vi "Proyecto Final_Topicos.vi"() -> ()   [LabVIEW 2020]
uses:
  <vilib>/Instr/_visa.llb/VISA Configure Serial Port (Instr).vi
  <vilib>/vision/NI_Vision_Development_Module.lvlib
panel:
  out "Buffer Completo":string
  out "Number of Particles":i32
  out "Particle Reports (Real-World)":T1(array[cluster]) {"Orientation" format="%.2f"; "Dimensions"."Height" format="%.2f"; "Dimensions"."Width" format="%.2f"; "Center of Mass"."Y" format="%.2f"; "Center of Mass"."X" format="%.2f"; "Bounding Rect"."Bottom" format="%.2f"; "Bounding Rect"."Right" format="%.2f"; "Bounding Rect"."Top" format="%.2f"; "Bounding Rect"."Left" format="%.2f"; "Number of Holes" format="%.2f"; "Area" format="%.2f"}
  in  "Tab Control":T2(tab)
  out "Original":T3(plugin-control) caption="Original Image"
  out "Threshold":T3(plugin-control) caption="Threshold Image"
  out "Fill Hole and Reject Border":T3(plugin-control) caption="Reject Border and Fill Holes"
  out "ROJO":bool
  out "VERDE":bool
  out "AMBAR":bool
  out "Área de particulas":T4(graph)
  out "Área de particualas total":dbl
  in  "name or relative path":path=path "C:/Users/axel2/Downloads/Proyecto Topicos/mexico_tmo_2013066_lrg.jpg"
  out "Valores House Keeping":T5
  out "Señales Analógicas":dynamicdata(graph)
  out "Señales Digitales":dynamicdata(graph)
  out "Buffer Filtrado":string
  out "error out":errorcluster
  in  "error in (no error)":errorcluster
  out "LISTO?":bool=TRUE
  in  "stop":bool
  in  "Comando":T6(ring)
  in  "Decisión":bool
  in  "VISA resource":refnum<visa-resource-name>="COM4"
  # "Variables del Satélite GXIBA"
  # "Comunicación con Satélite"
  # "Procesamiento de Riesgo Volcánico"
  # "SEMÁFORO VOLCÁNICO"
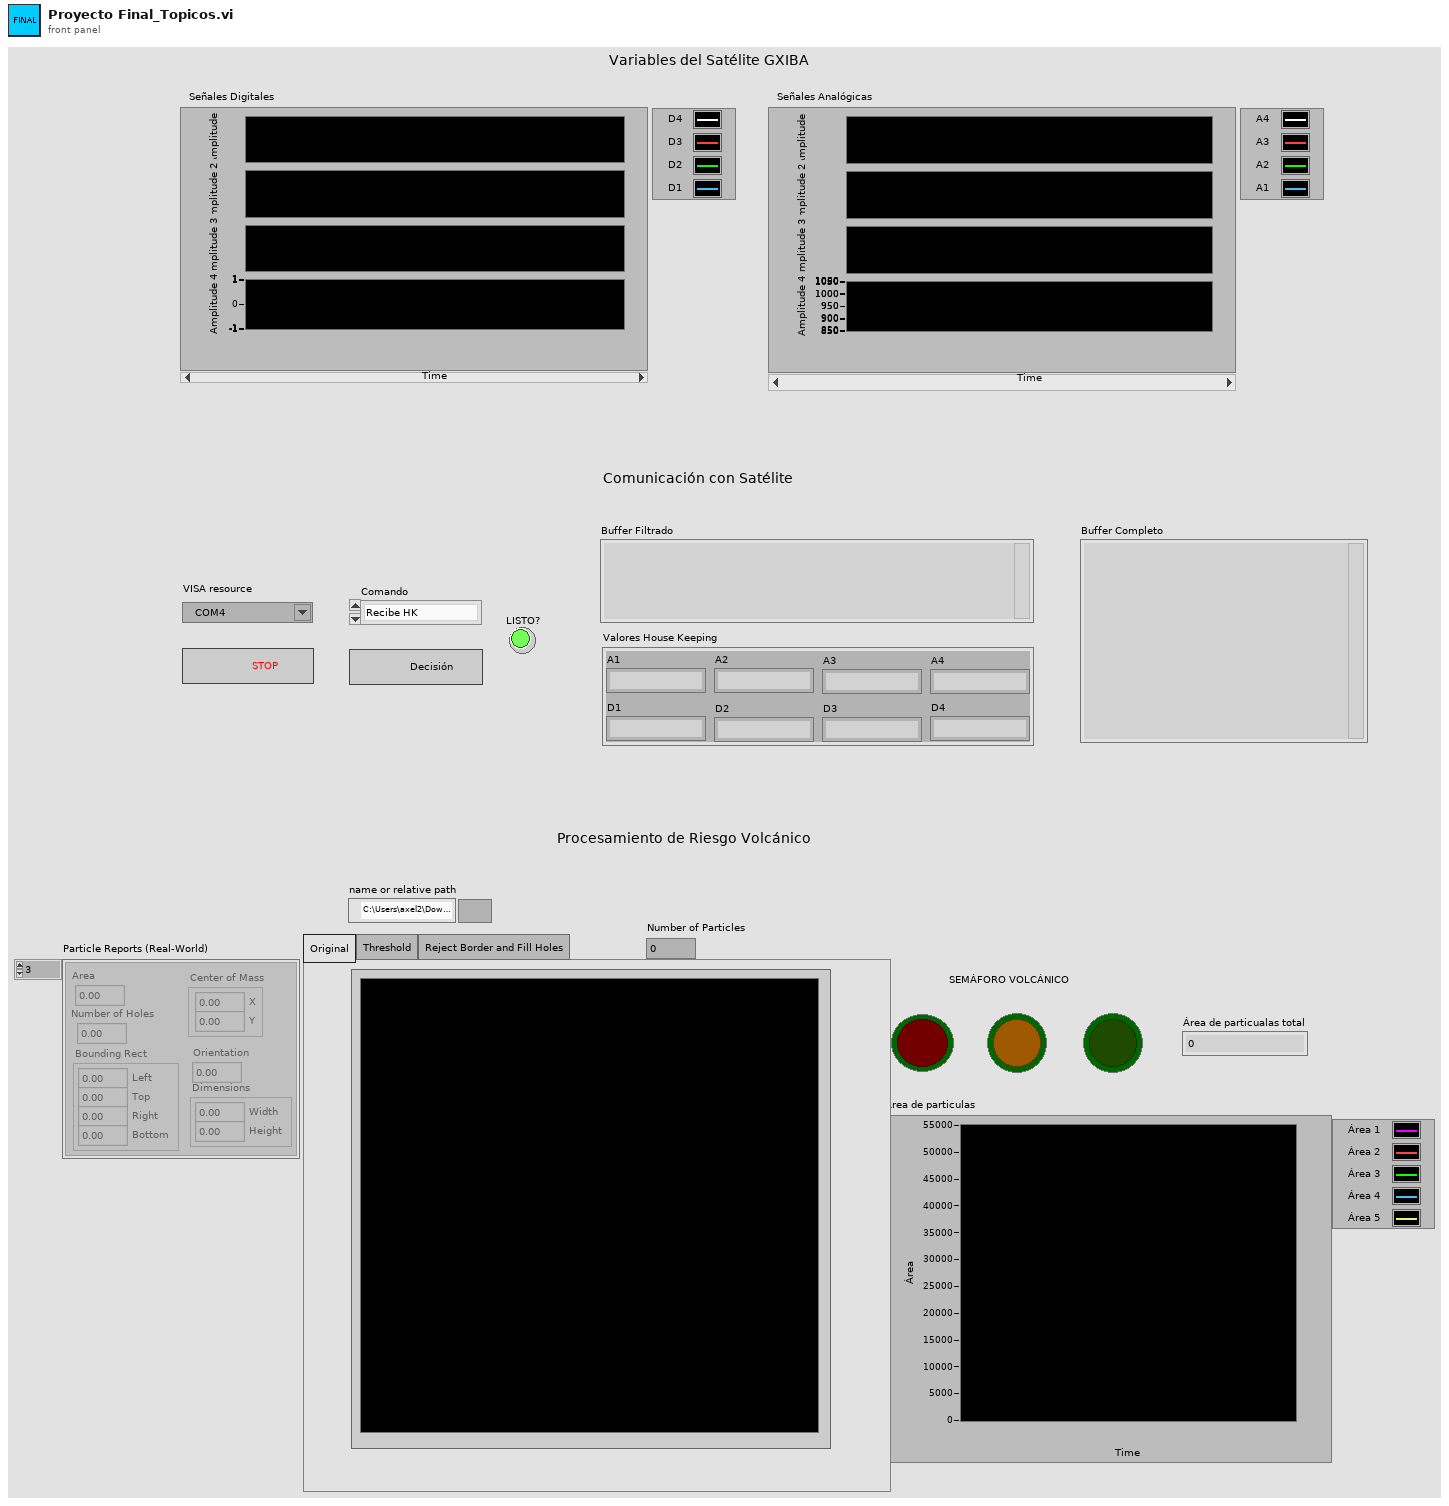
[diagram p1: front panel]
types:
  T1 = cluster{"Area":dbl, "Number of Holes":dbl, "Bounding Rect":cluster{"Left":dbl, "Top":dbl, "Right":dbl, "Bottom":dbl}, "Center of Mass":cluster{"X":dbl, "Y":dbl}, "Orientation":dbl, "Dimensions":cluster{"Width":dbl, "Height":dbl}}[]
  T2 = enum32{"Original", "Threshold", "Reject Border and Fill Holes"}
  T3 = typedef "IMAQ Image.ctl" = refnum<image>
  T4 = cluster{"Area":dbl, "Area":dbl, "Area":dbl, "Area":dbl, "Area":dbl}
  T5 = cluster{"A1":string, "A2":string, "A3":string, "A4":string, "D1":string, "D2":string, "D3":string, "D4":string}
  T6 = enum16{"Recibe HK", "Act Fecha", "Parametros", "Reset", "Stop"}
  T7 = typedef "Image Type" = u32
  T8 = cluster{"Particle Reports (Real-World)  [0]":cluster{"Area":dbl, "Number of Holes":dbl, "Bounding Rect":cluster{"Left":dbl, "Top":dbl, "Right":dbl, "Bottom":dbl}, "Center of Mass":cluster{"X":dbl, "Y":dbl}, "Orientation":dbl, "Dimensions":cluster{"Width":dbl, "Height":dbl}}, "Particle Reports (Real-World)  [1]":cluster{"Area":dbl, "Number of Holes":dbl, "Bounding Rect":cluster{"Left":dbl, "Top":dbl, "Right":dbl, "Bottom":dbl}, "Center of Mass":cluster{"X":dbl, "Y":dbl}, "Orientation":dbl, "Dimensions":cluster{"Width":dbl, "Height":dbl}}, "Particle Reports (Real-World)  [2]":cluster{"Area":dbl, "Number of Holes":dbl, "Bounding Rect":cluster{"Left":dbl, "Top":dbl, "Right":dbl, "Bottom":dbl}, "Center of Mass":cluster{"X":dbl, "Y":dbl}, "Orientation":dbl, "Dimensions":cluster{"Width":dbl, "Height":dbl}}, "Particle Reports (Real-World)  [3]":cluster{"Area":dbl, "Number of Holes":dbl, "Bounding Rect":cluster{"Left":dbl, "Top":dbl, "Right":dbl, "Bottom":dbl}, "Center of Mass":cluster{"X":dbl, "Y":dbl}, "Orientation":dbl, "Dimensions":cluster{"Width":dbl, "Height":dbl}}, "Particle Reports (Real-World)  [4]":cluster{"Area":dbl, "Number of Holes":dbl, "Bounding Rect":cluster{"Left":dbl, "Top":dbl, "Right":dbl, "Bottom":dbl}, "Center of Mass":cluster{"X":dbl, "Y":dbl}, "Orientation":dbl, "Dimensions":cluster{"Width":dbl, "Height":dbl}}, "Particle Reports (Real-World)  [5]":cluster{"Area":dbl, "Number of Holes":dbl, "Bounding Rect":cluster{"Left":dbl, "Top":dbl, "Right":dbl, "Bottom":dbl}, "Center of Mass":cluster{"X":dbl, "Y":dbl}, "Orientation":dbl, "Dimensions":cluster{"Width":dbl, "Height":dbl}}, "Particle Reports (Real-World)  [6]":cluster{"Area":dbl, "Number of Holes":dbl, "Bounding Rect":cluster{"Left":dbl, "Top":dbl, "Right":dbl, "Bottom":dbl}, "Center of Mass":cluster{"X":dbl, "Y":dbl}, "Orientation":dbl, "Dimensions":cluster{"Width":dbl, "Height":dbl}}, "Particle Reports (Real-World)  [7]":cluster{"Area":dbl, "Number of Holes":dbl, "Bounding Rect":cluster{"Left":dbl, "Top":dbl, "Right":dbl, "Bottom":dbl}, "Center of Mass":cluster{"X":dbl, "Y":dbl}, "Orientation":dbl, "Dimensions":cluster{"Width":dbl, "Height":dbl}}, "Particle Reports (Real-World)  [8]":cluster{"Area":dbl, "Number of Holes":dbl, "Bounding Rect":cluster{"Left":dbl, "Top":dbl, "Right":dbl, "Bottom":dbl}, "Center of Mass":cluster{"X":dbl, "Y":dbl}, "Orientation":dbl, "Dimensions":cluster{"Width":dbl, "Height":dbl}}}
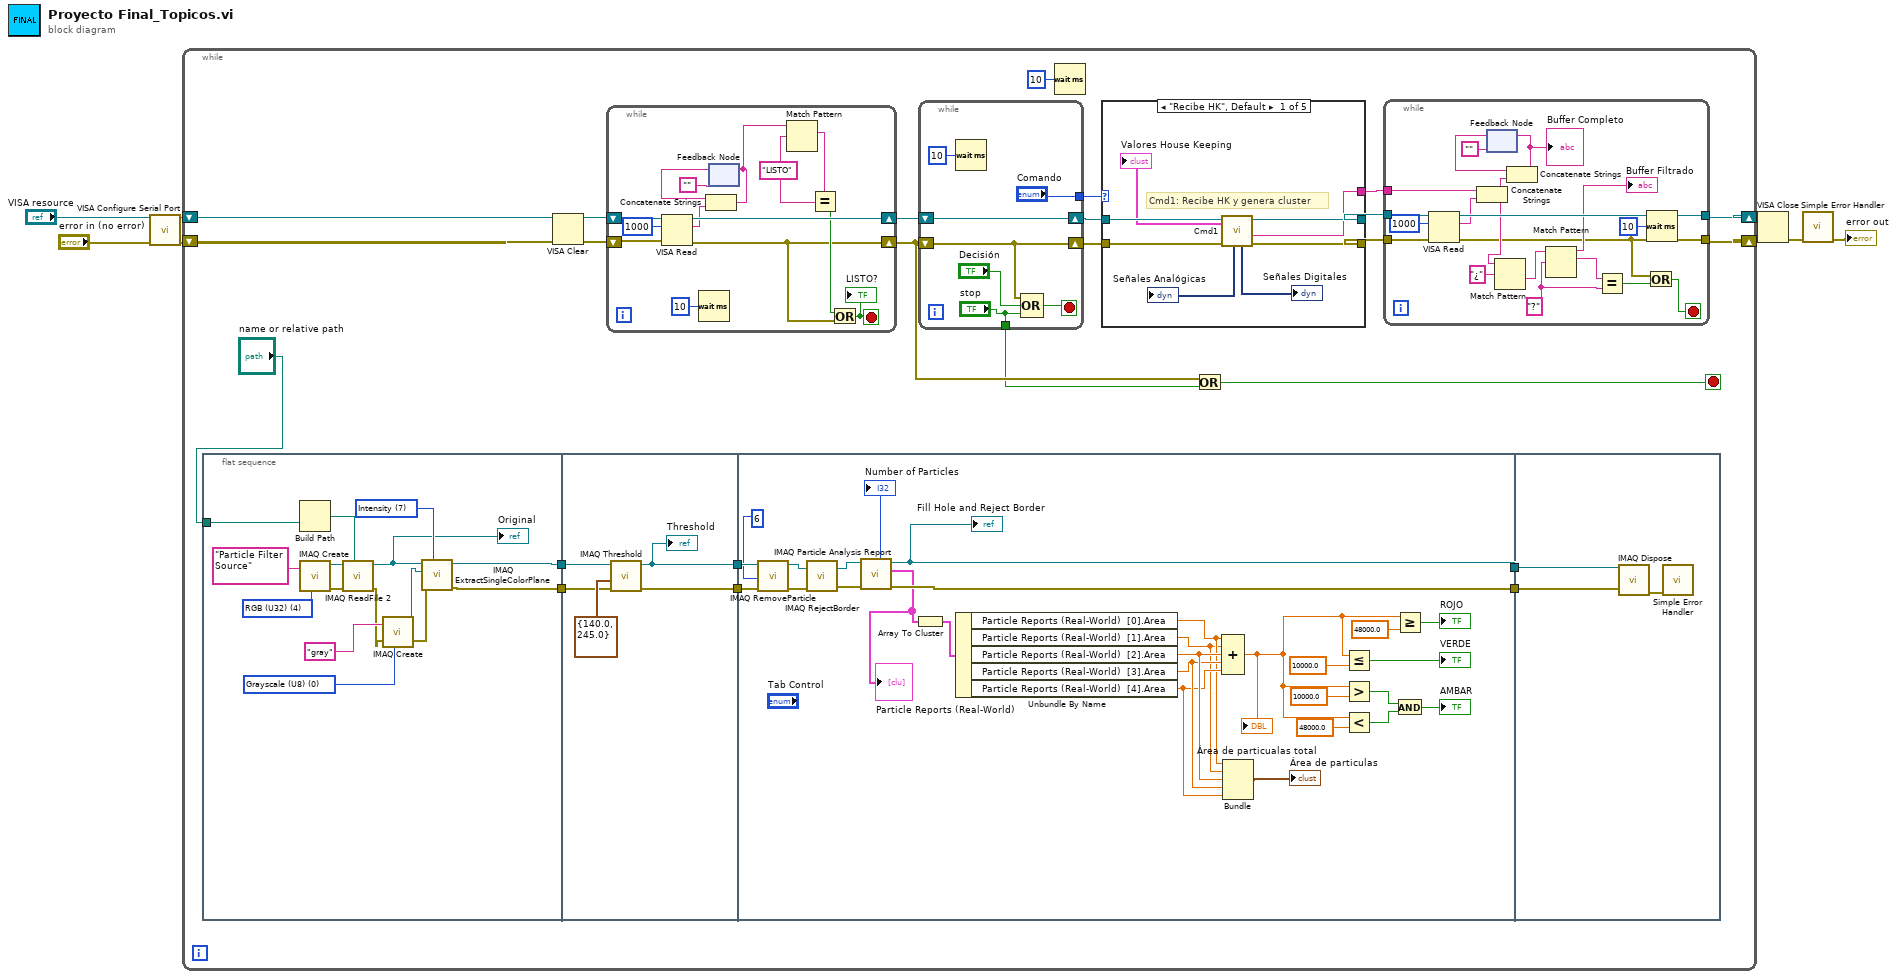
[diagram p0: block diagram]
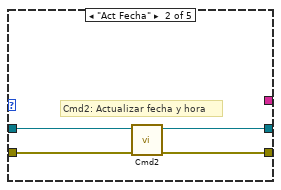
[diagram p2: hidden frame]
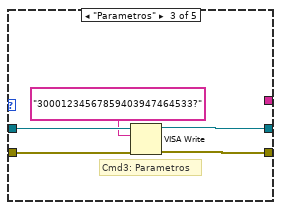
[diagram p3: hidden frame]
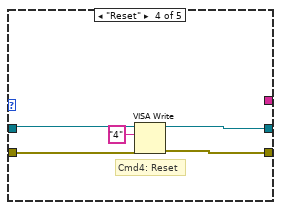
[diagram p4: hidden frame]
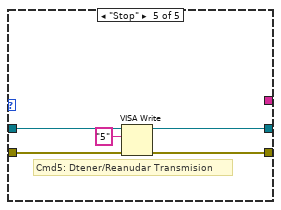
[diagram p5: hidden frame]
diagram:
  n1 = call-poly "VISA Configure Serial Port"("VISA resource name"="VISA resource", "error in (no error)"="error in (no error)") -> ("VISA resource name out"=w2:refnum<visa-resource-name>, "error out"=w1:errorcluster)  [unwired: 12 in]
  n2 = while {
    shift-right: [w19] -> w5
    shift-left: w1 -> [w25]
    shift-right: [w20] -> w6
    shift-left: w2 -> [w27]
    stop <- w28 stop-if-true
    n3 = flat-sequence {
      tunnel: [w35] -> w15
      tunnel: [w42] -> w14
      tunnel: "name or relative path" -> [w33]
      tunnel: [w50] -> w13
      tunnel: [w51] -> w12
      tunnel: w15 -> [w49]
      tunnel: w14 -> [w48]
      tunnel: w13 -> [w80]
      tunnel: w12 -> [w79]
      tunnel: [w54] -> w11
      tunnel: [w73] -> w10
      tunnel: w11 -> [w82]
      tunnel: w10 -> [w81]
      frame #0 {
        w39 = T7 0 items=["Grayscale (U8)", "Grayscale (I16)", "Grayscale (SGL)", "Complex (CSG)", "RGB (U32)", "HSL (U32)", "RGB (U64)", "Grayscale (U16)"] ("Image Type")
        w41 = 7 items=["Red", "Green", "Blue", "Hue", "Saturation", "Luminance", "Value", "Intensity"] ("Color Plane")
        w43 = T7 4 items=["Grayscale (U8)", "Grayscale (I16)", "Grayscale (SGL)", "Complex (CSG)", "RGB (U32)", "HSL (U32)", "RGB (U64)", "Grayscale (U16)"] ("Image Type")
        n4 = Build Path(name or relative path=w33) -> (appended path=w47:path)  [unwired: 1 in]
        n5 = call "IMAQ Create"("Image Name"="Particle Filter Source", "Image Type"=w43) -> ("New Image"=w45:T3, "error out"=w44:errorcluster)  [unwired: 3 in]
        n6 = call "IMAQ ReadFile 2"("File Path"=w47, "error in (no error)"=w44, "Image"=w45) -> ("error out"=w37:errorcluster, "Image Out"=w34:T3)  [unwired: 4 in, 3 out]
        "Original" <- w34
        n7 = call "IMAQ Create"("Image Name"="gray", "Image Type"=w39, "error in (no error)"=w37) -> ("New Image"=w40:T3, "error out"=w36:errorcluster)  [unwired: 2 in]
        n8 = call "IMAQ ExtractSingleColorPlane"("Color Plane"=w41, "error in (no error)"=w36, "Image Dst"=w40, "Image Src"=w34) -> ("error out"=w42:errorcluster, "Image Dst Out"=w35:T3)  [unwired: 6 in]
      }
      frame #1 {
        n9 = call "IMAQ Threshold"("error in (no error)"=w48, "Range"=cluster{"Lower value":sgl, "Upper value":sgl} {"Lower value"=140.0, "Upper value"=245.0}, "Image Src"=w49) -> ("error out"=w51:errorcluster, "Image Dst Out"=w50:T3)  [unwired: 7 in]
        "Threshold" <- w50
      }
      frame #2 {
        n10 = call "IMAQ RemoveParticle"("error in (no error)"=w79, "Number of Erosion"=6, "Image Src"=w80) -> ("error out"=w77:errorcluster, "Image Dst Out"=w78:T3)  [unwired: 7 in]
        n11 = call "IMAQ RejectBorder"("error in (no error)"=w77, "Image Src"=w78) -> ("error out"=w74:errorcluster, "Image Dst Out"=w75:T3)  [unwired: 4 in]
        n12 = call "IMAQ Particle Analysis Report"("error in (no error)"=w74, "Image"=w75) -> ("error out"=w73:errorcluster, "Particle Reports (Real-World)"=w53:T1, "Image Out (duplicate)"=w54:T3, "Number of Particles"=→"Number of Particles":i32)  [unwired: 6 out]
        "Fill Hole and Reject Border" <- w54
        "Particle Reports (Real-World)" <- w53
        n13 = Array To Cluster(array=w53) -> (cluster=w72:T8)
        n14 = Unbundle By Name(w72) -> ("Particle Reports (Real-World)  [0].Area"=w58:dbl, "Particle Reports (Real-World)  [1].Area"=w57:dbl, "Particle Reports (Real-World)  [2].Area"=w61:dbl, "Particle Reports (Real-World)  [3].Area"=w60:dbl, "Particle Reports (Real-World)  [4].Area"=w59:dbl)
        n15 = Compound Arithmetic op=ADD(w58, w57, w61, w60, w59) -> (w62:dbl)
        "Área de particualas total" <- w62
        n16 = Bundle("Area"=w58, "Area"=w57, "Area"=w61, "Area"=w60, "Area"=w59) -> (→"Área de particulas":T4)  [unwired: 1 in]
        n17 = Less Or Equal?(x=w62, y=10000.0) -> (x <= y?=→"VERDE":bool)
        n18 = Greater?(x=w62, y=10000.0) -> (0:w69:bool)
        n19 = Less?(x=w62, y=48000.0) -> (x < y?=w68:bool)
        n20 = Greater Or Equal?(x=w62, y=48000.0) -> (x >= y?=→"ROJO":bool)
        n21 = And(x=w69, y=w68) -> (x .and. y?=→"AMBAR":bool)
      }
      frame #3 {
        n22 = call "IMAQ Dispose"("Image"=w82, "error in (no error)"=w81) -> ("error out"=w83:errorcluster)  [unwired: 4 in]
        n23 = call <vilib>:"Simple Error Handler.vi"("error in (no error)"=w83) -> ()  [unwired: 4 in, 5 out]
      }
    }
    n24 = VISA Clear(VISA resource name=w27, error in (no error)=w25) -> (VISA resource name out=w26:refnum<visa-resource-name>, error out=w24:errorcluster)
    n25 = while {
      shift-right: [w138] -> w18
      shift-left: w24 -> [w149]
      shift-right: [w147] -> w30
      shift-left: w26 -> [w150]
      stop <- w137 stop-if-true
      w140 = "LISTO" ("regular expression")
      n26 = VISA Read(VISA resource name=w150, byte count=u32 1000, error in (no error)=w149) -> (VISA resource name out=w147:refnum<visa-resource-name>, read buffer=w146:string, error out=w138:errorcluster)  [unwired: 1 out]
      n27 = Wait (ms)(milliseconds to wait=u32 10) -> ()  [unwired: 1 out]
      n28 = feedback #1("") -> (w145:string)
      n29 = Concatenate Strings(w145, w146) -> (w142:string)
      n30 = feedback-in #1(w142) -> ()
      n31 = Match Pattern(string=w142, regular expression=w140) -> (match substring=w141:string)  [unwired: 1 in, 3 out]
      n32 = Equal?(x=w141, y=w140) -> (x = y?=w139:bool)
      n33 = Or(x=w139, y=w138) -> (x .or. y?=w137:bool)
      "LISTO?" <- w137
    }
    n34 = while {
      tunnel: ["Comando"] -> w32
      shift-right: [w108] -> w31
      shift-left: w30 -> [w108]
      shift-right: [w105] -> w29
      shift-left: w18 -> [w105]
      tunnel: ["stop"] -> w17
      stop <- w106 stop-if-true
      n35 = Wait (ms)(milliseconds to wait=u32 10) -> ()  [unwired: 1 out]
      n36 = Compound Arithmetic op=OR(w105, "Decisión", "stop") -> (w106:bool)
    }
    n37 = Wait (ms)(milliseconds to wait=u32 10) -> ()  [unwired: 1 out]
    n38 = case shown="\"Recibe HK\", Default" w32 {
      tunnel: w31 -> [w117 w121 w124 w131 w136]
      tunnel: w29 -> [w116 w120 w123 w130 w134]
      tunnel: [w114 w119 w126 w128 w135] -> w22
      tunnel: [w115 w118 w125 w129 w133] -> w21
      tunnel: [w113 _ _ _ _] -> w16
      frame "Recibe HK", Default {
        # "Cmd1: Recibe HK y genera cluster"
        n39 = call "Cmd1.vi"("error in (no error)"=w116, "VISA Refnum in"=w117) -> ("error out (no error)"=w115:errorcluster, "read buffer"=w113:string, "VISA Refnum in 2"=w114:refnum<visa-resource-name>, "Señales Digitales"=→"Señales Digitales":dynamicdata, "Señales Analógicas"=→"Señales Analógicas":dynamicdata, "Señales"=→"Valores House Keeping":T5)  [unwired: 4 in]
      }
      frame "Act Fecha" {
        # "Cmd2: Actualizar fecha y hora"
        n40 = call "Cmd2.vi"("error in (no error)"=w120, "VISA Refnum in"=w121) -> ("error out"=w118:errorcluster, "VISA Refnum out"=w119:refnum<visa-resource-name>)  [unwired: 7 in, 1 out]
      }
      frame "Parametros" {
        # "Cmd3: Parametros"
        n41 = VISA Write(VISA resource name=w124, write buffer="30001234567859403947464533?", error in (no error)=w123) -> (VISA resource name out=w126:refnum<visa-resource-name>, error out=w125:errorcluster)  [unwired: 1 out]
      }
      frame "Reset" {
        # "Cmd4: Reset"
        n42 = VISA Write(VISA resource name=w131, write buffer="4", error in (no error)=w130) -> (VISA resource name out=w128:refnum<visa-resource-name>, error out=w129:errorcluster)  [unwired: 1 out]
      }
      frame "Stop" {
        # "Cmd5: Dtener/Reanudar Transmision"
        n43 = VISA Write(VISA resource name=w136, write buffer="5", error in (no error)=w134) -> (VISA resource name out=w135:refnum<visa-resource-name>, error out=w133:errorcluster)  [unwired: 1 out]
      }
    }
    n44 = Or(x=w18, y=w17) -> (x .or. y?=w28:bool)
    n45 = while {
      tunnel: w22 -> [w100]
      tunnel: w21 -> [w99]
      tunnel: [w95] -> w20
      tunnel: [w85] -> w19
      tunnel: w16 -> [w87]
      stop <- w84 stop-if-true
      w96 = "?" ("regular expression")
      n46 = VISA Read(VISA resource name=w100, byte count=u32 1000, error in (no error)=w99) -> (VISA resource name out=w95:refnum<visa-resource-name>, read buffer=w92:string, error out=w85:errorcluster)  [unwired: 1 out]
      n47 = Concatenate Strings(w87, w92) -> (w91:string)
      n48 = feedback #2("") -> (w89:string)
      n49 = Match Pattern(string=w91, regular expression="¿") -> (after substring=w101:string)  [unwired: 1 in, 3 out]
      n50 = Concatenate Strings(w89, w91) -> (w90:string)
      "Buffer Completo" <- w90
      n51 = feedback-in #2(w90) -> ()
      n52 = Match Pattern(string=w101, regular expression=w96) -> (before substring=→"Buffer Filtrado":string, match substring=w94:string)  [unwired: 1 in, 2 out]
      n53 = Equal?(x=w94, y=w96) -> (x = y?=w86:bool)
      n54 = Or(x=w85, y=w86) -> (x .or. y?=w84:bool)
      n55 = Wait (ms)(milliseconds to wait=u32 10) -> ()  [unwired: 1 out]
    }
  }
  n56 = VISA Close(VISA resource name=w6, error in (no error)=w5) -> (error out=w8:errorcluster)
  n57 = call <vilib>:"Simple Error Handler.vi"("error in (no error)"=w8) -> ("error out"=→"error out":errorcluster)  [unwired: 4 in, 4 out]
